vi "Directional Speed Run Test.vi"() -> ()   [LabVIEW 2015]
uses:
  IP Source/Directional Speed/Input.ctl
  IP Source/Directional Speed/Settings.ctl
  IP Source/APU/Shared Settings.ctl
  IP Source/APU/Input.ctl
  IP Source/Directional Speed/Load Input.ctl
  <vilib>/rvi/interface/RandomDataEmulation/nirviRandomDataOpen.vi
  <vilib>/rvi/interface/common/niFpgaCacheSessionInfoDynamic.vi
  <vilib>/Utility/error.llb/Error Cluster From Error Code.vi
  <vilib>/rvi/errors/niLvFpgaAdjustHostInterfaceError.vi
  <vilib>/FPGAPlugInAG/Dynamic/niLvFpga_Run_Dynamic.vi
  <vilib>/FPGAPlugInAG/Dynamic/niLvFpga_Close_Dynamic.vi
  <vilib>/rvi/interface/nirviOpenFPGA/nirviOpenFPGA.xnode
  Compile Tests/APU + 1 Directional Sim.vi
  <vilib>/rvi/interface/nirviReadWriteControl/nirviReadWriteControl.xnode
  <vilib>/rvi/interface/nirviMethod/nirviMethod.xnode
  <vilib>/rvi/interface/nirviCloseFPGA/nirviCloseFPGA.xnode
  <vilib>/rvi/interface/Simulation/niFpgaSimulationCallBeginRW.vi
  IP Source/APU/APU.lvlib
  NiFpgaLv.dll
  IP Source/Directional Speed/Directional Speed.lvlib
  IP Source/Engine Simulation Toolkit.lvlib
panel:
  in  "Starting Crank Angle":u16
  in  "direction speed inputs":T1={"td (tics)"=200, "tf (tics)"=1800, "tr (tics)"=3600}
  in  "Tooth Centers":u16[](array[numeric])=[18204, 36408, 54613]
  out "Load done":bool
  out "Load time (s)":dbl
  in  "RPM":dbl=5000.0 format="%#_15g"
  in  "stop":bool
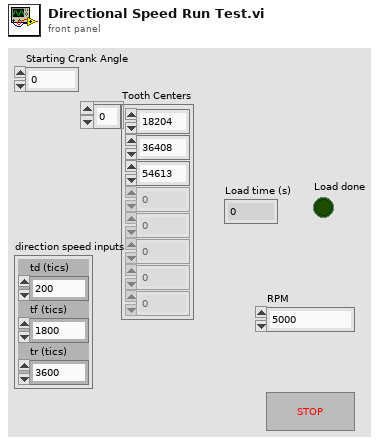
[diagram p1: front panel]
types:
  T1 = typedef "Engine Simulation Toolkit.lvlib/Directional Speed.lvlib/Input.ctl" = cluster{"td (tics)":u16, "tf (tics)":u16, "tr (tics)":u16}
  T2 = typedef "Engine Simulation Toolkit.lvlib/APU.lvlib/Shared Settings.ctl" = cluster{"start":fxp<+,17,17>, "stuck limit":fxp<+,18,18>}
  T3 = typedef "Engine Simulation Toolkit.lvlib/Directional Speed.lvlib/Settings.ctl" = cluster{"Upper Value":u16, "Lower Value":u16, "Upper Index":fxp<+,10,10>, "Lower Index":fxp<+,10,10>, "Enabled":bool}
  T4 = typedef "Engine Simulation Toolkit.lvlib/Directional Speed.lvlib/Load Input.ctl" = cluster{"address":fxp<+,10,10>, "done":bool, "angle":u16}
  T5 = typedef "Engine Simulation Toolkit.lvlib/APU.lvlib/Input.ctl" = cluster{"desired speed":fxp<+/-,23,2>, "reset":bool}
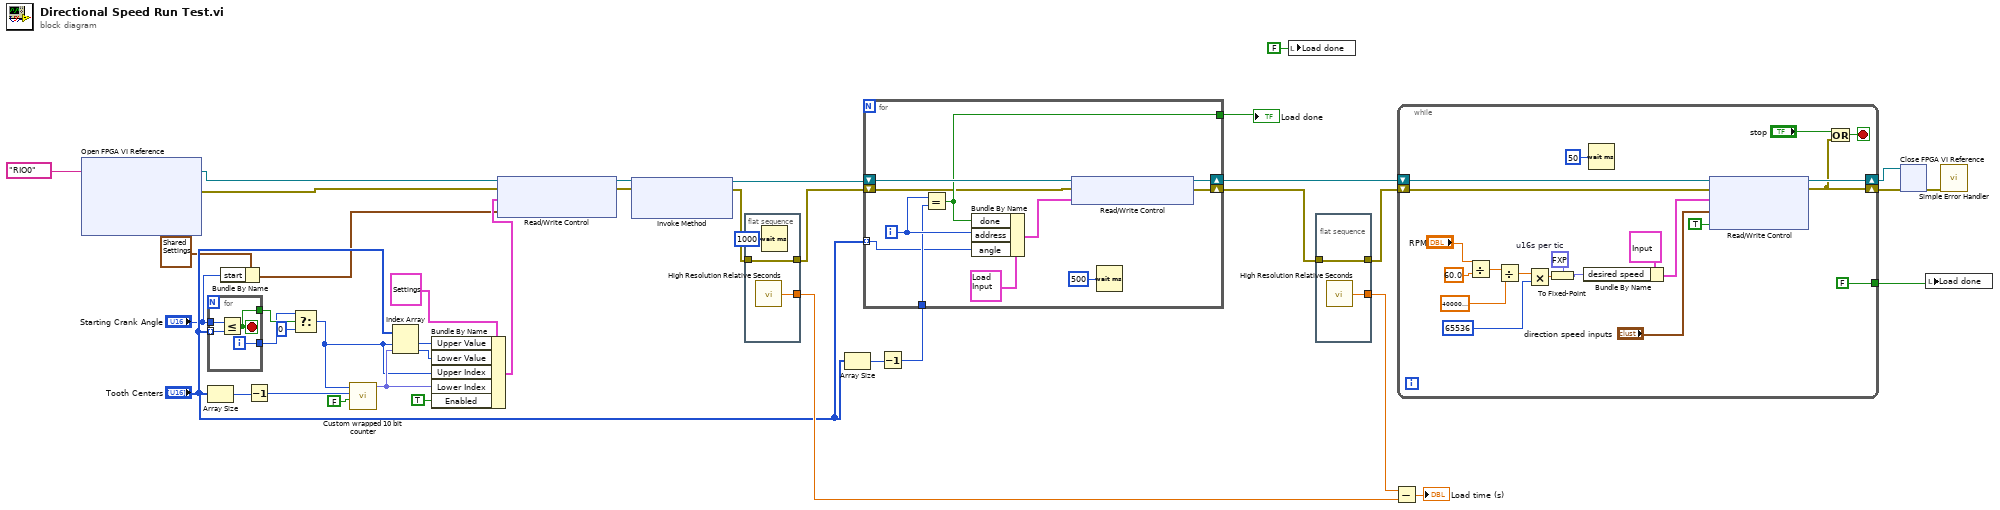
[diagram p0: block diagram]
diagram:
  n1 = xnode "Open FPGA VI Reference"("resource name"=tag "RIO0") -> ("FPGA VI Reference Out"=w18:refnum<k20>, "error out"=w36:errorcluster)  [unwired: 1 in]
  n2 = for {
    tunnel: "Starting Crank Angle" -> [w43]
    tunnel: "Tooth Centers" -> [w42] mode=indexing
    tunnel: [w41] -> w3
    tunnel: [w40] -> w4
    i -> [w41]
    stop <- w40 stop-if-true
    n3 = Less Or Equal?(x=w43, y=w42) -> (x <= y?=w40:bool)
  }
  n4 = Array Size(array="Tooth Centers") -> (size(s)=w17:i32)
  n5 = Bundle By Name(cluster=T2 {"start"=0.0, "stuck limit"=0.0} ("APU Shared Settings"), "start"="Starting Crank Angle") -> (w6:T2)
  n6 = Decrement(x=w17) -> (x-1=w13:i32)
  n7 = Select(t=w3, s=w4, f=0) -> (s? t:f=w1:i32)
  n8 = call "Custom wrapped 10 bit counter.vi"("increment or decrement (decrement)"=FALSE, "max value"=w13, "value"=w1) -> ("new value"=w12:fxp<+,10,10>)  [unwired: 7 in, 1 out]
  n9 = Index Array(array="Tooth Centers", index #1=w1, index #2=w12) -> (element #1=w11:u16, element #2=w10:u16)
  n10 = Bundle By Name(cluster=T3 {"Upper Value"=0, "Lower Value"=0, "Upper Index"=0.0, "Lower Index"=0.0, "Enabled"=FALSE} ("settings.<user name>"), "Upper Value"=w11, "Lower Value"=w10, "Upper Index"=w1, "Lower Index"=w12, "Enabled"=TRUE) -> (w9:T3)
  n11 = xnode "Read/Write Control"("FPGA VI Reference In"=w18, "error in"=w36, "settings.DirectionSim"=w9, "shared settings.my apu"=w6) -> ("FPGA VI Reference Out"=w22:refnum<k20>, "error out"=w23:errorcluster)
  n12 = xnode "Invoke Method"("FPGA VI Reference In"=w22, "error in"=w23) -> ("FPGA VI Reference Out"=w32:refnum<k20>, "error out"=w30:errorcluster)  [unwired: 1 in]
  n13 = flat-sequence {
    tunnel: [w46] -> w31
    tunnel: w30 -> [w46]
    tunnel: [w45] -> w28
    frame #0 {
      n14 = call <vilib>:"High Resolution Relative Seconds.vi"() -> ("relative seconds"=w45:dbl)
      n15 = Wait (ms)(milliseconds to wait=u32 1000) -> ()  [unwired: 1 out]
    }
  }
  n16 = Array Size(array="Tooth Centers") -> (size(s)=w21:i32)
  n17 = Decrement(x=w21) -> (x-1=w20:i32)
  n18 = for {
    shift-right: [w54] -> w25
    shift-left: w31 -> [w48]
    shift-right: [w56] -> w26
    shift-left: w32 -> [w57]
    tunnel: "Tooth Centers" -> [w47] mode=indexing
    tunnel: w20 -> [w51]
    tunnel: [w49] -> w19
    i -> [w52]
    n19 = Equal?(x=w52, y=w51) -> (x = y?=w49:bool)
    n20 = Bundle By Name(cluster=T4 {"address"=0.0, "done"=FALSE, "angle"=0} ("load input.<user name>"), "done"=w49, "address"=w52, "angle"=w47) -> (w50:T4)
    n21 = xnode "Read/Write Control"("FPGA VI Reference In"=w57, "error in"=w48, "load input.DirectionSim"=w50) -> ("FPGA VI Reference Out"=w56:refnum<k20>, "error out"=w54:errorcluster)
    n22 = Wait (ms)(milliseconds to wait=u32 500) -> ()  [unwired: 1 out]
  }
  "Load done" <- w19
  n23 = local write "Load done"(FALSE ("Load done")) -> ()
  n24 = flat-sequence {
    tunnel: [w59] -> w24
    tunnel: w25 -> [w59]
    tunnel: [w58] -> w29
    frame #0 {
      n25 = call <vilib>:"High Resolution Relative Seconds.vi"() -> ("relative seconds"=w58:dbl)
    }
  }
  n26 = Subtract(x=w29, y=w28) -> (x-y=→"Load time (s)":dbl)
  n27 = while {
    shift-right: [w75] -> w39
    shift-left: w24 -> [w80]
    shift-right: [w78] -> w38
    shift-left: w26 -> [w79]
    tunnel: [FALSE ("Load")] -> w34
    stop <- w76 stop-if-true
    w68 = fxp<+/-,23,2> 0.0  # u16s per tic
    n28 = Divide(x="RPM", y=60.0) -> (x/y=w72:dbl)
    n29 = Divide(x=w72, y=40000000.0) -> (x/y=w69:dbl)
    n30 = Multiply(x=w69, y=u32 65536 ("n")) -> (x*y=w67:dbl)
    n31 = To Fixed-Point(fixed-point type=w68, number=w67) -> (fixed-point=w63:fxp<+/-,23,2>)
    n32 = Bundle By Name(cluster=T5 {"desired speed"=0.0, "reset"=FALSE} ("my apu"), "desired speed"=w63) -> (w62:T5)
    n33 = Wait (ms)(milliseconds to wait=u32 50) -> ()  [unwired: 1 out]
    n34 = xnode "Read/Write Control"("FPGA VI Reference In"=w79, "error in"=w80, "input.my apu"=w62, "input.DirectionSim"="direction speed inputs", "go.my apu"=TRUE) -> ("FPGA VI Reference Out"=w78:refnum<k20>, "error out"=w75:errorcluster)
    n35 = Or(x="stop", y=w75) -> (x .or. y?=w76:bool)
  }
  n36 = xnode "Close FPGA VI Reference"("FPGA VI Reference In"=w38, "error in"=w39) -> ("error out"=w37:errorcluster)
  n37 = local write "Load done"(w34) -> ()
  n38 = call <vilib>:"Simple Error Handler.vi"("error in (no error)"=w37) -> ()  [unwired: 4 in, 5 out]
